vi "Get UI Details.vi"() -> ()   [LabVIEW 2020, in "Keysight 34401A DMM Measurement.lvlib"]
uses:
  Keysight 34401A DMM Measurement.lvlib
  <vilib>/Plug-In SDKs/Measurements/Helpers/TypeDefs/User Interface Information.ctl
  <vilib>/Plug-In SDKs/Measurements/NI Measurement Plug-In SDK.lvlib
panel:
  out "error out":errorcluster
  in  "error in (no error)":errorcluster
  out "user interface details":T1[](array[typedef])
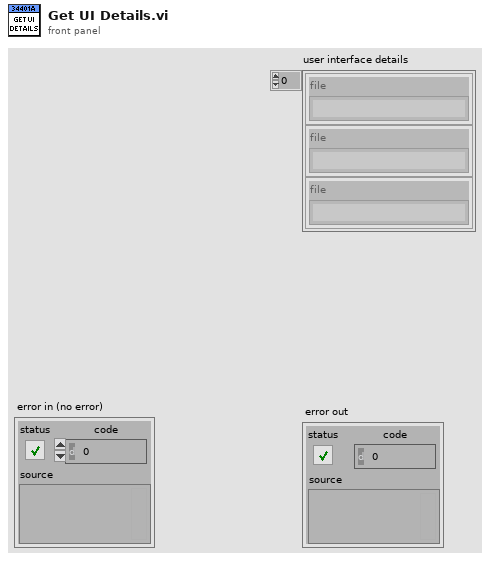
[diagram p1: front panel]
types:
  T1 = typedef "NI Measurement Plug-In SDK.lvlib/User Interface Information.ctl" = cluster{"file":string}
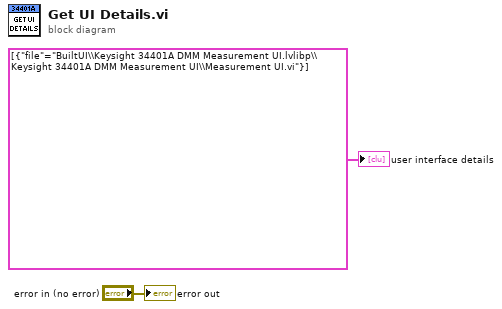
[diagram p0: block diagram]
diagram:
  "user interface details" <- T1[] [{"file"="BuiltUI\\Keysight 34401A DMM Measurement UI.lvlibp\\Keysight 34401A DMM Measurement UI\\Measurement UI.vi"}] ("appended array")
  "error out" <- "error in (no error)"
